vi "Tester.vi"(8 "error in (no error)":errorcluster, 9 "Default":T1, 11 "Tag Name":string) -> (0 "error out":errorcluster, 1 "Value":T1)   [LabVIEW 2010]
doc: "This VI will read the data associated with a single tag. This VI will always look up the tag index if the name changes, or if index lookup failed previously (resulting in an error). This combines the functionality of the CVT2 VIs for reads and static reads."
uses:
  Type Defs/Memory Commands.ctl
  Current Value Table.lvlib
  FGVs/Tag Index Memory Methods.ctl
  DataTypes/I32_Memory Block.vi
  DataTypes/I32_Type To Enum.vi
  DataTypes/Template_Datatype.ctl
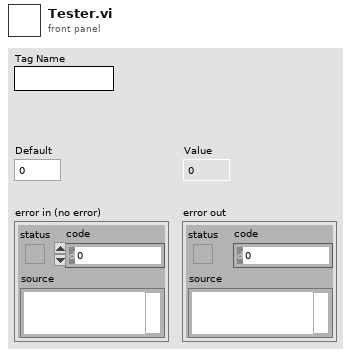
[diagram p1: front panel]
types:
  T1 = typedef "Current Value Table.lvlib/Template_Datatype.ctl" = i32
  T2 = typedef "Current Value Table.lvlib/Tag Index Memory Methods.ctl" = enum16{"Clear", "Set Tag Index", "Read Tag Index", "Set Tag Indices", "Read Tag Indices", "Check Existence"}
  T3 = typedef "Current Value Table.lvlib/Index Types.ctl" = cluster{"Data Type":T4, "Index":i32}
  T4 = typedef "Current Value Table.lvlib/Data Types.ctl" = enum16{"Double", "Single", "I64", "I32", "I16", "I8", "Boolean", "String", "U8", "U16", "U32", "U64"}
  T5 = typedef "Current Value Table.lvlib/Data Types.ctl" = enum16{"Single", "Double", "Boolean", "I8", "I16", "I32", "I64", "U8", "U16", "U32", "U64", "String"}
  T6 = typedef "Current Value Table.lvlib/Memory Commands.ctl" = enum16{"Init", "Add Data", "Read", "Read Group", "Read All", "Write", "Write Group", "Get Size"}
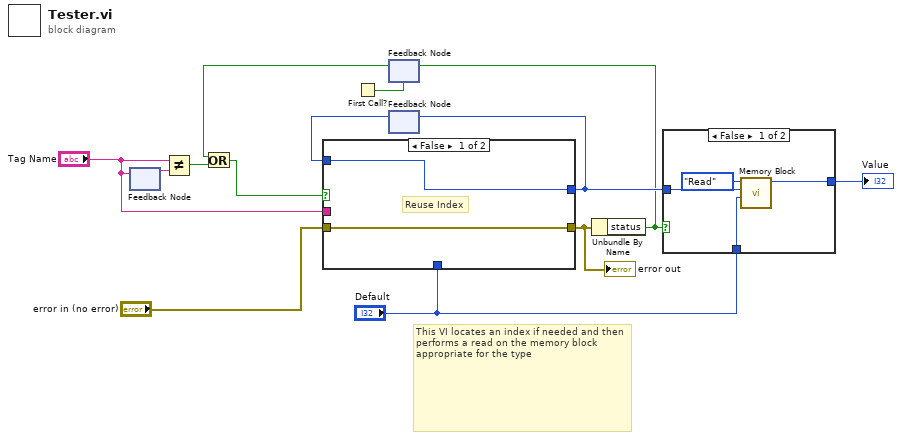
[diagram p0: block diagram]
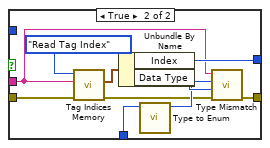
[diagram p3: hidden frame]
diagram:
  # "This VI locates an index if needed and then performs a read on the memory block appropriate for the type"
  n1 = feedback #1() -> (w12:string)  [unwired: 1 in]
  n2 = feedback-in #1("Tag Name") -> ()
  n3 = Not Equal?(x="Tag Name", y=w12) -> (x != y?=w5:bool)
  n4 = First Call?() -> (First Call?: T/F=w1:bool)
  n5 = feedback #2(w1) -> (w3:bool)
  n6 = Or(x=w3, y=w5) -> (x .or. y?=w2:bool)
  n7 = feedback #3() -> (w11:i32)  [unwired: 1 in]
  n8 = case shown="False" w2 {
    tunnel: [w15 w25] -> w6
    tunnel: "error in (no error)" -> [w15 w24]
    tunnel: [w14 w20] -> w10
    tunnel: w11 -> [w14 _]
    tunnel: "Default" -> [_ w16]
    tunnel: "Tag Name" -> [_ w19]
    frame False {
      # "Reuse Index"
    }
    frame True {
      n9 = call "Tag Indices Memory.vi"("error in (no error)"=w24, "Tag"=w19, "Method"=Tag_Index_Memory_Methods."Read Tag Index") -> ("error out"=w17:errorcluster, "Index Type Out"=w22:T3)  [unwired: 6 in, 1 out]
      n10 = Unbundle By Name(w22) -> ("Index"=w20:i32, "Data Type"=w21:T4)
      n11 = call-poly "Type to Enum.vi"("Default"=w16) -> ("Data Type Enum"=w18:T5)  [unwired: 10 in]
      n12 = call "Type Mismatch.vi"("error in (no error)"=w17, "Data Type Requested"=w21, "True Type"=w18, "Tag"=w19) -> ("error out"=w25:errorcluster)  [unwired: 7 in]
    }
  }
  "error out" <- w6
  n13 = feedback-in #3(w10) -> ()
  n14 = Unbundle By Name(w6) -> ("status"=w4:bool)
  n15 = feedback-in #2(w4) -> ()
  n16 = case shown="False" w4 {
    tunnel: w10 -> [w28 _]
    tunnel: "Default" -> [w27 w30]
    tunnel: [w26 w30] -> w7
    frame False {
      n17 = call-poly "Memory Block.vi"("Value"=w27, "Index"=w28, "Method"=Memory_Commands."Read") -> ("Value Out"=w26:i32)  [unwired: 6 in, 2 out]
    }
    frame True {
    }
  }
  "Value" <- w7
